vi "SerializeSliceCalc.vi"(8 "error in (no error)":errorcluster, 10 "Options":T1, 11 "Class to Serialize":refnum<class "BlueSerializable.lvclass">) -> (0 "error out":errorcluster, 2 "All class layers":T3[](array[typedef]), 3 "Class to Serialize":refnum<class "BlueSerializable.lvclass">)   [LabVIEW 2019, in "BlueSerialization.lvlib" / "BlueSerializer.lvclass"]
uses:
  BlueSerializer.lvclass
  BlueSerializable/BlueSerializable.lvclass
  Support/GetSerializableDataClusterClass.ctl
  Support/SerializableDataGetDataAction.ctl
  ClassNameAndVersion.ctl
  <vilib>/Utility/EditLVLibs/LibVersion.ctl
  SerializeOptionsPayload.ctl
  SerializeOptions.ctl
  ClassNameCacheMap.ctl
  ClassNameObj.ctl
  Support/GetParentClassesHiererchy.vi
  ClassNameCacheWrite.vi
  GetLastCompatibleVersion.vi
  <userlib>/_OpenG.lib/lvdata/lvdata.llb/LVOOP Get Default Object__ogtk.vi
  <vilib>/Utility/LVClass/Get LV Class Name.vi
  <vilib>/Utility/LVClass/Get LV Class Default Value By Name.vi
  <vilib>/Utility/EditLVLibs/LVClass/Get Mutation History.vi
  <vilib>/Utility/error.llb/Error Cluster From Error Code.vi
  <vilib>/Utility/EditLVLibs/Edit LVLibs.lvlib
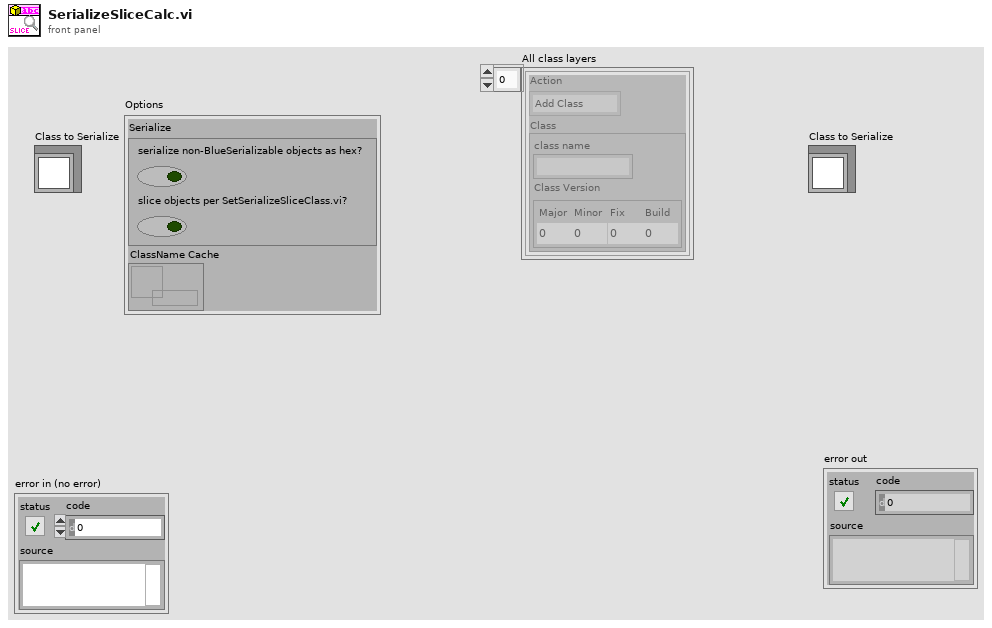
[diagram p1: front panel]
types:
  T1 = typedef "BlueSerialization.lvlib/BlueSerializer.lvclass/SerializeOptionsPayload.ctl" = cluster{"Serialize":T2, "ClassName Cache":refnum<data-value>}
  T2 = typedef "BlueSerialization.lvlib/BlueSerializer.lvclass/SerializeOptions.ctl" = cluster{"serialize non-BlueSerializable objects as hex?":bool, "slice objects per SetSerializeSliceClass.vi?":bool}
  T3 = typedef "BlueSerialization.lvlib/BlueSerializer.lvclass/GetSerializableDataClusterClass.ctl" = cluster{"Action":T4, "Class":T5}
  T4 = typedef "BlueSerialization.lvlib/BlueSerializer.lvclass/SerializableDataGetDataAction.ctl" = enum16{"Add Class", "Drop Class"}
  T5 = typedef "BlueSerialization.lvlib/BlueSerializer.lvclass/ClassNameAndVersion.ctl" = cluster{"class name":string, "Class Version":T6}
  T6 = typedef "Edit LVLibs.lvlib/LibVersion.ctl" = cluster{"Major":u16, "Minor":u16, "Fix":u16, "Build":u16}
  T7 = typedef "BlueSerialization.lvlib/BlueSerializer.lvclass/ClassNameObj.ctl" = cluster{"class name":string, "default object":refnum<class>}
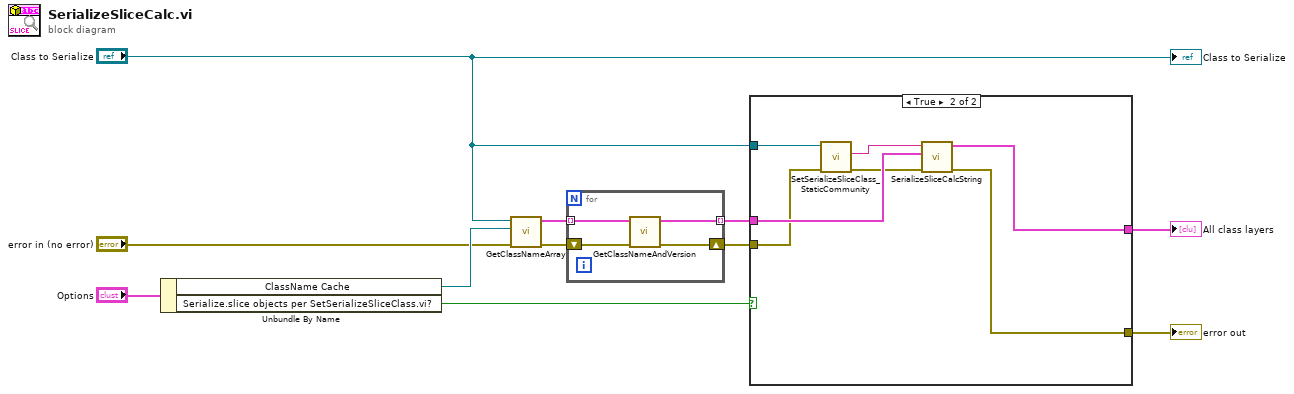
[diagram p0: block diagram]
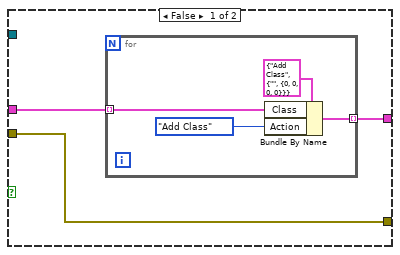
[diagram p2: hidden frame]
diagram:
  n1 = Unbundle By Name("Options") -> ("ClassName Cache"=w10:refnum<data-value>, "Serialize.slice objects per SetSerializeSliceClass.vi?"=w8:bool)
  n2 = call "GetClassNameArray.vi"("error in (no error)"="error in (no error)", "ClassName Cache"=w10, "LabVIEW Object in"="Class to Serialize") -> ("error out"=w2:errorcluster, "Class (child,parent)"=w4:T7[])  [unwired: 7 in]
  n3 = for {
    tunnel: w4 -> [w15] mode=indexing
    tunnel: [w13] -> w3 mode=indexing
    shift-right: [w12] -> w1
    shift-left: w2 -> [w14]
    n4 = call "GetClassNameAndVersion.vi"("error in (no error)"=w14, "Class"=w15) -> ("error out"=w12:errorcluster, "Class NameVer"=w13:T5)  [unwired: 8 in]
  }
  n5 = case shown="True" w8 {
    tunnel: "Class to Serialize" -> [_ w26]
    tunnel: w3 -> [w18 w29]
    tunnel: [w17 w27] -> w5
    tunnel: [w16 w28] -> w6
    tunnel: w1 -> [w16 w25]
    frame False {
      n6 = for {
        tunnel: w18 -> [w19] mode=indexing
        tunnel: [w20] -> w17 mode=indexing
        n7 = Bundle By Name(cluster=T3 {"Action"=enum."Add Class", "Class"={"class name"="", "Class Version"={"Major"=0, "Minor"=0, "Fix"=0, "Build"=0}}} ("Cluster 2"), "Class"=w19, "Action"=SerializableDataGetDataAction."Add Class") -> (w20:T3)
      }
    }
    frame True {
      n8 = call "SetSerializeSliceClass_StaticCommunity.vi"("error in (no error)"=w25, "BlueSerializable in"=w26) -> ("error out"=w24:errorcluster, "Slice-To-This Class Name"=w23:string)  [unwired: 8 in]
      n9 = call "SerializeSliceCalcString.vi"("error in (no error)"=w24, "Class NameVer"=w29, "Slice-To-This Class Name"=w23) -> ("error out"=w28:errorcluster, "Class"=w27:T3[])  [unwired: 7 in]
    }
  }
  "All class layers" <- w5
  "error out" <- w6
  "Class to Serialize" <- "Class to Serialize"
